vi "Compass Begin.vi"(2 "Port Number":u8, 3 "error in (no error)":errorcluster, 4 "Address":u16=33, 5 "FPGA VI Reference":T1) -> (0 "error out":errorcluster, 1 "FPGA Information Out":T2)   [LabVIEW 2012, in "Compass IO.lvlib"]
uses:
  Compass IO.lvlib
  <vilib>/IEDriver/SPIandI2C/Host/I2C/I2C Host.lvlib
  FPGA_ref.ctl
panel:
  in  "Address Type (7-bit)":enum16{"7-bit", "10-bit"}(ring)
  in  "Clock Rate":u32=1000
  in  "FPGA Clock (40 MHz)":u32=40000000
  # "Compass I2C interface\n=====\nInitialize compass communication and set to Continuous Read @ 20Hz.\nHeading can then be read out using Compass Read block.\nDefault ettings below should work in all cases."
  # "Default port 0"
  # "Compass address: 33 dec ( 0x42 >> 1 )"
  # "7-bit"
  # "1Khz clock"
  # "40MHz FPGA clock"
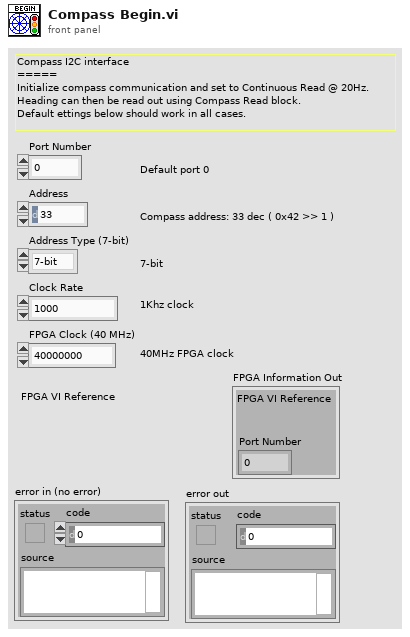
[diagram p1: front panel]
types:
  T1 = typedef "FPGA_ref.ctl" = refnum<k20>
  T2 = cluster{"FPGA VI Reference":T1, "Port Number":u8}
  T3 = cluster{"FPGA VI Reference":refnum<k20>, "Port Number":u8}
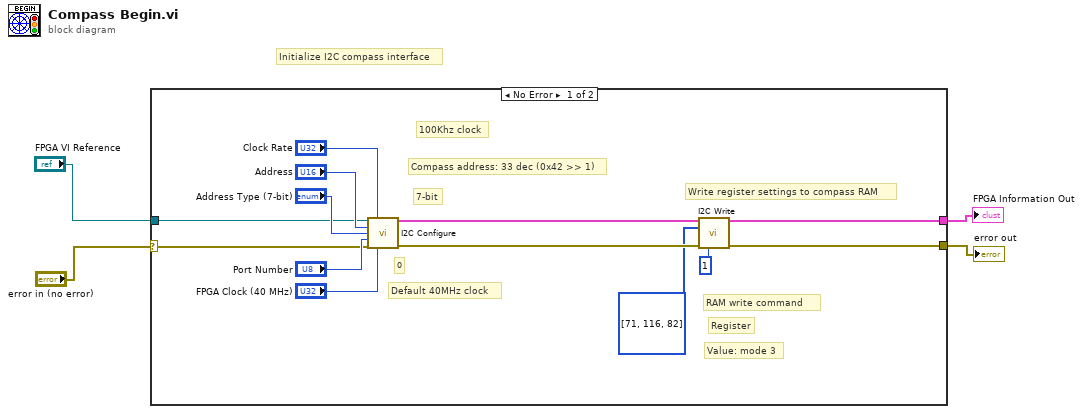
[diagram p0: block diagram]
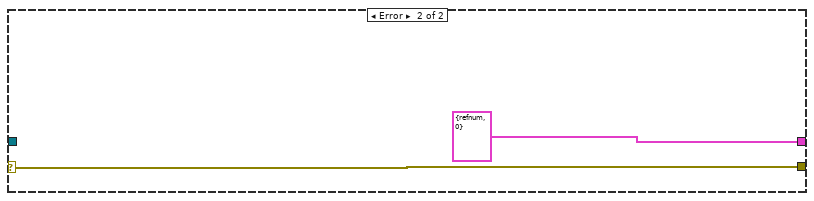
[diagram p2: hidden frame]
diagram:
  # "Initialize I2C compass interface"
  n1 = case shown="No Error" "error in (no error)" {
    selector: "error in (no error)" -> [w11 w19]
    tunnel: "FPGA VI Reference" -> [w12 _]
    tunnel: [w8 T3 {"FPGA VI Reference"=refnum, "Port Number"=0} ("FPGA Information Out")] -> w3
    tunnel: [w7 w19] -> w2
    frame No Error {
      # "Value: mode 3"
      # "Register"
      # "RAM write command"
      # "Write register settings to compass RAM"
      # "100Khz clock"
      # "0"
      # "7-bit"
      # "Compass address: 33 dec (0x42 >> 1)"
      # "Default 40MHz clock"
      n2 = call <vilib>:"I2C Configure.vi"("FPGA VI Reference"=w12, "Clock Rate"="Clock Rate", "Address"="Address", "Address Type (7-bit)"="Address Type (7-bit)", "Port Number"="Port Number", "error in (no error)"=w11, "FPGA Clock (40 MHz)"="FPGA Clock (40 MHz)") -> ("FPGA Information Out"=w10:T3, "error out"=w9:errorcluster)  [unwired: 7 in]
      n3 = call <vilib>:"I2C Write.vi"("FPGA Information In"=w10, "Data"=u8[] [71, 116, 82], "error in (no error)"=w9, "Timeout (10 s)"=u8 1) -> ("FPGA Information Out"=w8:T3, "error out"=w7:errorcluster)  [unwired: 10 in]
    }
    frame Error {
    }
  }
  "FPGA Information Out" <- w3
  "error out" <- w2
